vi "Configure RF Upconversion.vi"(7 "User Defined Frequency (1.95GHz)":dbl=1950000000.0 format="%#.9p", 8 "error in (no error)":errorcluster, 9 "Phase Compensation (Off)":i32(ring) items=["Off", "Carrier Frequency", "User Defined"], 10 "Instance (1)":T1=1, 11 "VISA resource name":refnum<visa-resource-name>) -> (0 "error out":errorcluster, 3 "VISA resource name out":refnum<visa-resource-name>)   [LabVIEW 2020, in "Rohde&Schwarz CMWXP NR FR1 Measurement.lvlib"]
doc: "Specifies the phase compensation applied by the UE during the modulation and upconversion.\n\nAttribute:\nRSCMWXPNRFR1M_ATTR_RF_UPCONVERSION\n\nRemote-control command:\nCONFigure:NRSub:MEAS<i>:MEValuation:PCOMp"
uses:
  <instrlib>/Rohde&Schwarz CMWXP NR FR1 Measurement/Rohde&Schwarz CMWXP NR FR1 Measurement.lvlib
  <instrlib>/Rohde&Schwarz CMWXP NR FR1 Measurement/Private/_Instance.ctl
  <instrlib>/Rohde&Schwarz CMWXP NR FR1 Measurement/Private/rsidr_core.llb/rsidr_core.lvlib
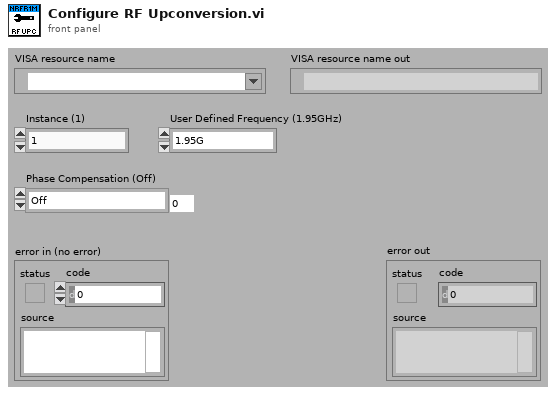
[diagram p1: front panel]
types:
  T1 = typedef "Rohde&Schwarz CMWXP NR FR1 Measurement.lvlib/_Instance.ctl" = i32
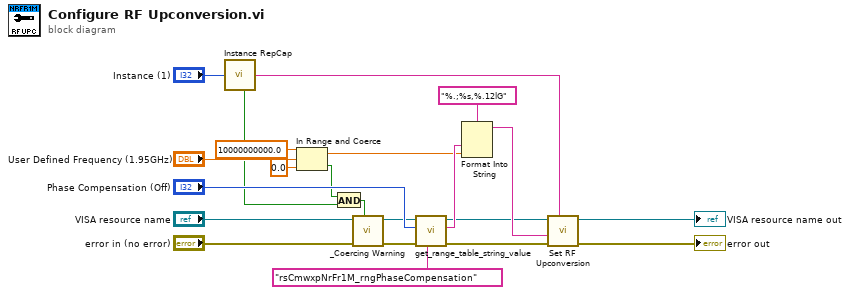
[diagram p0: block diagram]
diagram:
  n1 = call <instrlib>:"Instance RepCap.vi"("Instance In"="Instance (1)") -> ("In Range?"=w2:bool, "RepCap Identifier Out"=w17:string)  [unwired: 1 in]
  n2 = In Range and Coerce(upper limit=10000000000.0, x="User Defined Frequency (1.95GHz)", lower limit=0.0) -> (coerced(x)=w6:dbl, In Range?=w1:bool)
  n3 = And(x=w1, y=w2) -> (x .and. y?=w3:bool)
  n4 = call <instrlib>:"_Coercing Warning.vi"("In Range?"=w3, "error in (no error)"="error in (no error)", "VISA resource name"="VISA resource name") -> ("error out"=w9:errorcluster, "VISA resource name out"=w8:refnum<visa-resource-name>)  [unwired: 7 in]
  n5 = call <instrlib>:"get_range_table_string_value.vi"("Range Table ID in"="rsCmwxpNrFr1M_rngPhaseCompensation", "error in"=w9, "I32 input"="Phase Compensation (Off)", "VISA resource name"=w8) -> ("error out"=w12:errorcluster, "String Value out"=w15:string, "VISA resource name out"=w13:refnum<visa-resource-name>)  [unwired: 5 in]
  n6 = Format Into String(format string="%.;%s,%.12lG", w15, w6) -> (resulting string=w14:string)  [unwired: 2 in, 1 out]
  n7 = call "Set RF Upconversion"("Repeated Capabilities"=w17, "error in (no error)"=w12, "RF Upconversion ()"=w14, "instrument handle"=w13) -> ("error out"=→"error out":errorcluster, "instrument handle out"=→"VISA resource name out":refnum<visa-resource-name>)  [unwired: 6 in]
